vi "AWS_DataFinder_PrepareDataFinder.vi"(8 "error in":errorcluster, 11 "DataFinder":T1="My DataFinder") -> (0 "error out":errorcluster, 3 "DataFinder reference out":T1)   [LabVIEW 2014]
doc: "Optimize custom properties to run the example queries with high performance."
uses:
  <vilib>/userdefined/High Color/DFDataFinder.ctl
  <vilib>/DataFinder/DataTypes/object type.ctl
  <vilib>/DataFinder/DataTypes/property.ctl
  <vilib>/DataFinder/DataTypes/data type.ctl
  <vilib>/DataFinder/NI_DataFinder Toolkit.lvlib
  <resource>/objmgr/DataFinder.rc
  <vilib>/userdefined/NI_DataFinder Controls.lvlib
panel:
  # "To run the DataFinder_Pass_Fail_Analysis example correctly some custom properties have to be optimized."
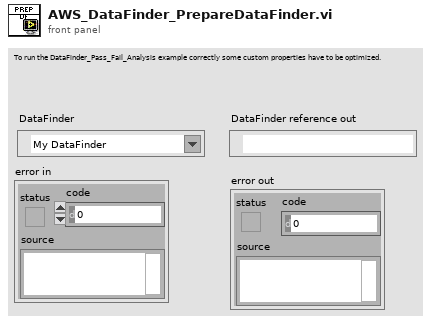
[diagram p1: front panel]
types:
  T1 = typedef "NI_DataFinder Controls.lvlib/DFDataFinder.ctl" = refnum<k21>
  T2 = typedef "NI_DataFinder Toolkit.lvlib/data type.ctl" = u16
  T3 = typedef "NI_DataFinder Toolkit.lvlib/property.ctl" = cluster{"object type":T4, "property name":string, "data type":T2}
  T4 = typedef "NI_DataFinder Toolkit.lvlib/object type.ctl" = u16
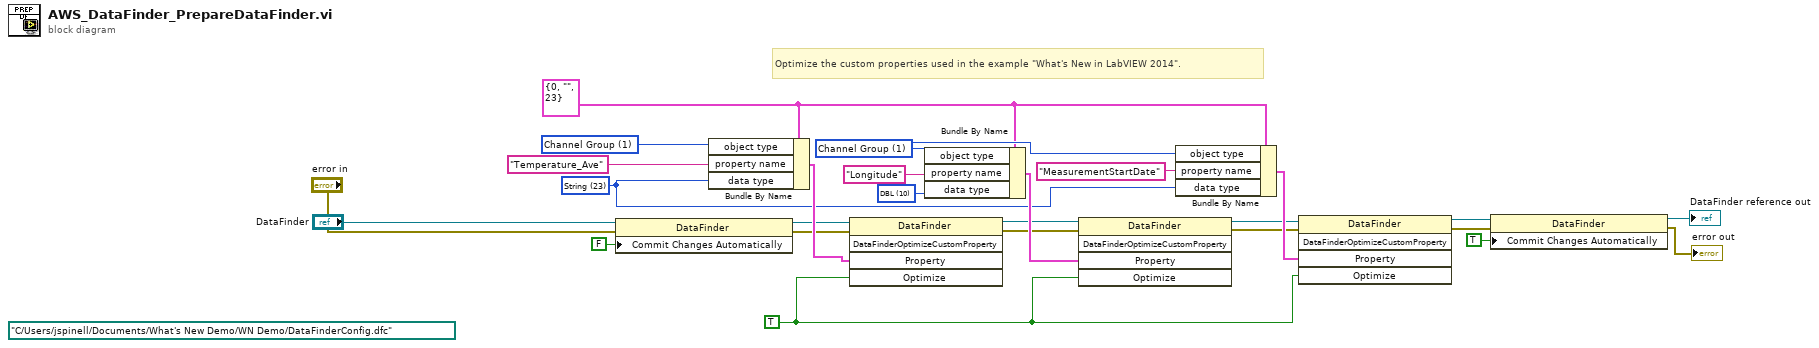
[diagram p0: block diagram]
diagram:
  (unwired) path "C:/Users/jspinell/Documents/What's New Demo/WN Demo/DataFinderConfig.dfc" ("Import File Path")
  w3 = T2 10 items=["Unknown"=0, "String"=23, "I32"=3, "DBL"=10, "Time stamp"=30] ("data type")
  w12 = T2 23 items=["Unknown"=0, "String"=23, "I32"=3, "DBL"=10, "Time stamp"=30] ("data type")
  w21 = T3 {"object type"=0, "property name"="", "data type"=23} ("property")
  w23 = T4 1 items=["File", "Channel Group", "Channel"] ("object type")
  w26 = T4 1 items=["File", "Channel Group", "Channel"] ("object type")
  w18 = TRUE ("optimize")
  # "Optimize the custom properties used in the example \"What's New in LabVIEW 2014\"."
  n1 = property class="DataFinder"(reference="DataFinder", error in="error in", "Commit Changes Automatically"=FALSE ("Settings:Commit Changes Automatically")) -> (reference out=w11:T1, error out=w7:errorcluster)
  n2 = Bundle By Name(cluster=w21, "object type"=w26, "property name"="Temperature_Ave", "data type"=w12) -> (w20:T3)
  n3 = invoke class="DataFinder" method="DataFinderOptimizeCustomProperty"(reference=w11, error in=w7, "Property"=w20, "Optimize"=w18) -> (reference out=w16:T1, error out=w15:errorcluster)  [unwired: 1 in, 3 out]
  n4 = Bundle By Name(cluster=w21, "object type"=w23, "property name"="Longitude", "data type"=w3) -> (w17:T3)
  n5 = invoke class="DataFinder" method="DataFinderOptimizeCustomProperty"(reference=w16, error in=w15, "Property"=w17, "Optimize"=w18) -> (reference out=w13:T1, error out=w14:errorcluster)  [unwired: 1 in, 3 out]
  n6 = Bundle By Name(cluster=w21, "object type"=w23, "property name"="MeasurementStartDate", "data type"=w12) -> (w19:T3)
  n7 = invoke class="DataFinder" method="DataFinderOptimizeCustomProperty"(reference=w13, error in=w14, "Property"=w19, "Optimize"=w18) -> (reference out=w6:T1, error out=w4:errorcluster)  [unwired: 1 in, 3 out]
  n8 = property class="DataFinder"(reference=w6, error in=w4, "Commit Changes Automatically"=TRUE ("Settings:Commit Changes Automatically")) -> (reference out=→"DataFinder reference out":T1, error out=→"error out":errorcluster)
